vi "Sensors_EV3.vi"   [LabVIEW 2012]
uses:
  SubVIs/LVPresent_Globals.vi
panel:
  # "Sensors\n\nThe EV3 comes with 5 sensors. These sensors enable the robot to perform many more tasks. The sensors are as follows:"
  # "ÊColor Sensor- can detect up to \n7 colors or a lack of a color, and \ncan detect light and its intensityÊ"
  # "Infrared Sensor- Can detect other robots\n within 50- 70 cm and signals up to 2 \nmeters away by the EV3 Infrared Beacon."
  # "Gyro Sensor- determine the rotation \nand orientation of the robot on several axes"
  # "Ultrasonic Sensor- emits sound waves in\norder to detect the distance from an object\nupto 250 cm, with an accuracy of +/- 1 cm"
  # "Touch Sensor- has a button on the front, \nand can detect press and release actions"
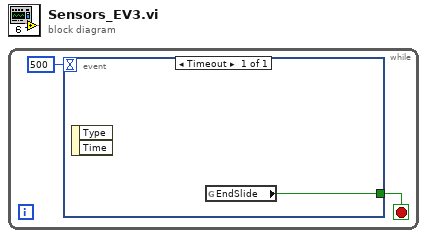
[diagram p0: block diagram]
diagram:
  n1 = while {
    stop <- w2 stop-if-true
    n2 = event shown="[0] Timeout" {
      selector: _ -> [_]
      dyn-events: _ -> [_]
      timeout: 500 -> [_]
      tunnel: [w3] -> w2
      event Timeout {
        n3 = event-data() -> ()  [unwired: 1 in, 2 out]
        n4 = global read "LVPresent_Globals.vi" "EndSlide"() -> (w3:bool)
      }
    }
  }
